vi "PPG_ABC.ProcEvents.vi"(0 "i ref in":refnum<vi>, 5 "error in (no error)":errorcluster) -> (14 "i ref out":refnum<vi>, 19 "error out":errorcluster)   [LabVIEW 2014, in "PPG_ABC.lvlib"]
doc: "This method is used to define the events the object will listen to. Add your own events here."
uses:
  PPG_ABC.lvlib
  CS_Core/BaseProcess/BaseProcess.event definition.ctl
  CS_Core/CAEObj/CAEObj.event definition.ctl
  CS_Core/BaseProcess/BaseProcess.descriptor string definition.ctl
  CS_Core/BaseProcess/BaseProcess.lvlib
  CS_Core/CAEObj/CAEObj.lvlib
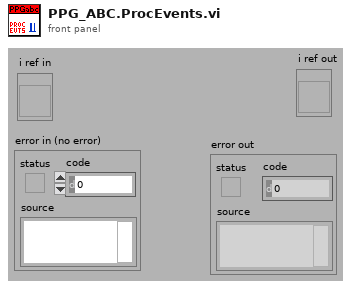
[diagram p1: front panel]
types:
  T1 = typedef "BaseProcess.lvlib/BaseProcess.event definition.ctl" = cluster{"CAEEvtDef":T2, "Data Descriptor":T3}
  T2 = typedef "CAEObj.lvlib/CAEObj.event definition.ctl" = cluster{"URL":string, "enable":bool, "ignoreResID":bool}
  T3 = typedef "BaseProcess.lvlib/BaseProcess.descriptor string definition.ctl" = string
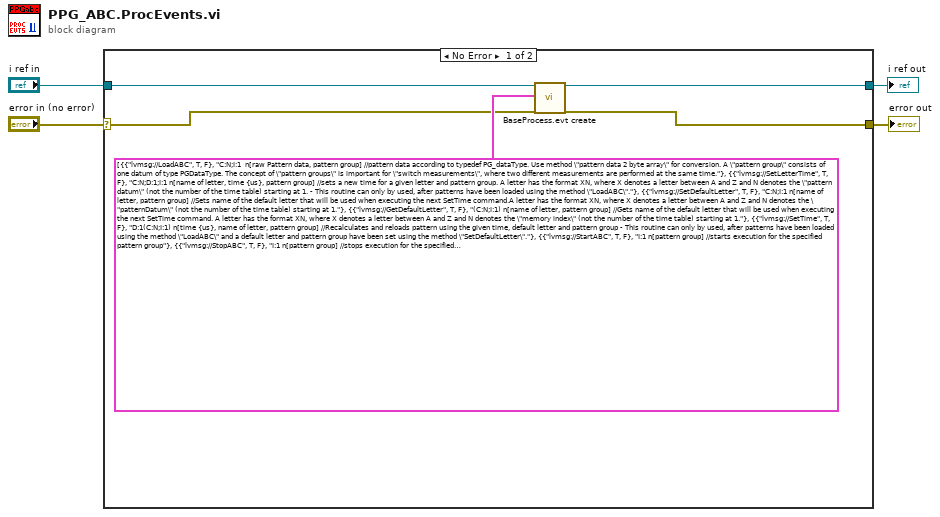
[diagram p0: block diagram]
diagram:
  n1 = case shown="No Error" "error in (no error)" {
    selector: "error in (no error)" -> [w5 w10]
    tunnel: "i ref in" -> [w9 w11]
    tunnel: [w8 w11] -> w3
    tunnel: [w7 w10] -> w2
    frame No Error {
      n2 = call "BaseProcess.evt create.vi"("i ref in"=w9, "newEvents"=T1[] [{"CAEEvtDef"={"URL"="lvmsg://LoadABC", "enable"=TRUE, "ignoreResID"=FALSE}, "Data Descriptor"="C:N;I:1  n[raw Pattern data, pattern group] //pattern data according to typedef PG_dataType. Use method \"pattern data 2 byte array\" for conversion. A \"pattern group\" consists of one datum of type PGDataType. The concept of \"pattern groups\" is important for \"switch measurements\", where two different measurements are performed at the same time."}, {"CAEEvtDef"={"URL"="lvmsg://SetLetterTime", "enable"=TRUE, "ignoreResID"=FALSE}, "Data Descriptor"="C:N;D:1;I:1 n[name of letter, time {us}, pattern group] //sets a new time for a given letter and pattern group. A letter has the format XN, where X denotes a letter between A and Z and N denotes the \"pattern datum\" (not the number of the time table) starting at 1. - This routine can only by used, after patterns have been loaded using the method \"LoadABC\"."}, {"CAEEvtDef"={"URL"="lvmsg://SetDefaultLetter", "enable"=TRUE, "ignoreResID"=FALSE}, "Data Descriptor"="C:N;I:1 n[name of letter, pattern group] //Sets name of the default letter that will be used when executing the next SetTime command.A letter has the format XN, where X denotes a letter between A and Z and N denotes the \"patternDatum\" (not the number of the time table) starting at 1."}, {"CAEEvtDef"={"URL"="lvmsg://GetDefaultLetter", "enable"=TRUE, "ignoreResID"=FALSE}, "Data Descriptor"="(C:N;I:1) n[name of letter, pattern group] //Gets name of the default letter that will be used when executing the next SetTime command. A letter has the format XN, where X denotes a letter between A and Z and N denotes the \"memory index\" (not the number of the time table) starting at 1."}, {"CAEEvtDef"={"URL"="lvmsg://SetTime", "enable"=TRUE, "ignoreResID"=FALSE}, "Data Descriptor"="D:1(C:N;I:1) n[time {us}, name of letter, pattern group] //Recalculates and reloads pattern using the given time, default letter and pattern group - This routine can only by used, after patterns have been loaded using the method \"LoadABC\" and a default letter and pattern group have been set using the method \"SetDefaultLetter\"."}, {"CAEEvtDef"={"URL"="lvmsg://StartABC", "enable"=TRUE, "ignoreResID"=FALSE}, "Data Descriptor"="I:1 n[pattern group] //starts execution for the specified pattern group"}, {"CAEEvtDef"={"URL"="lvmsg://StopABC", "enable"=TRUE, "ignoreResID"=FALSE}, "Data Descriptor"="I:1 n[pattern group] //stops execution for the specified pattern group"}] ("new events"), "error in (no error)"=w5) -> ("i ref out"=w8:refnum<vi>, "error out"=w7:errorcluster)  [unwired: 13 in, 2 out]
    }
    frame Error {
    }
  }
  "i ref out" <- w3
  "error out" <- w2
